vi "GV pixel count.vi"() -> ()   [LabVIEW 2017]
panel:
  out "Pixel count":u16
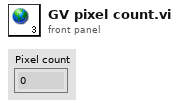
[diagram p1: front panel]
diagram:
